vi "Choreo_TrajectoryCacheDifferential_Clear.vi"(8 "error in (no error)":errorcluster) -> (0 "error out":errorcluster)   [LabVIEW 2019, in "ChoreoLib.lvlib"]
doc: "Clear the swerve memory cache\n\nInputs:\n -- ErrorIn -- cluster -- standard error cluster. Can be used to force execution sequence.\n\nOutputs:\n -- ErrorOut -- cluster -- standard error cluster. Can be used to force execution sequence and check for error."
uses:
  Choreo_Choreo_Globals.vi
  ChoreoLib.lvlib
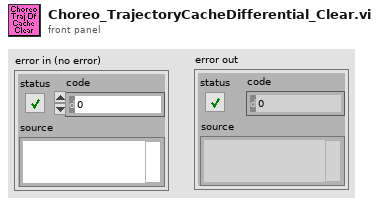
[diagram p1: front panel]
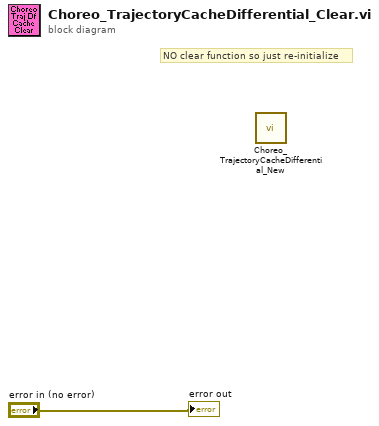
[diagram p0: block diagram]
diagram:
  # "NO clear function so just re-initialize"
  n1 = call "Choreo_TrajectoryCacheDifferential_New.vi"() -> ()  [unwired: 11 in, 1 out]
  "error out" <- "error in (no error)"
